vi "GetInstance.vi"(8 "error in (no error)":errorcluster, 11 "Singleton in":refnum<class "Singleton.lvclass">) -> (0 "error out":errorcluster, 3 "Singleton out":refnum<class "Singleton.lvclass">)   [LabVIEW 2014]
uses:
  Singleton.lvclass
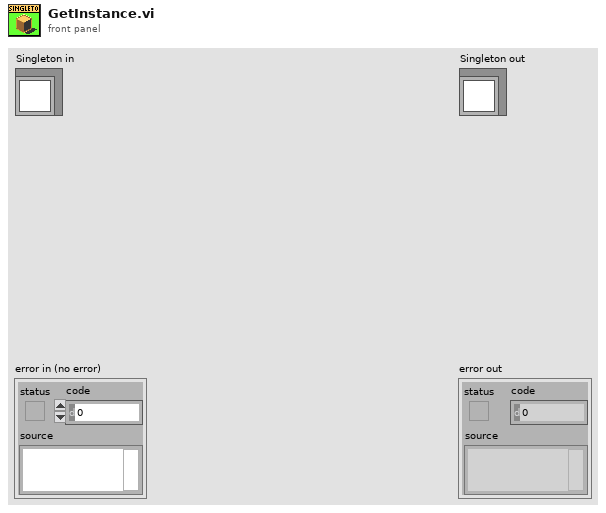
[diagram p1: front panel]
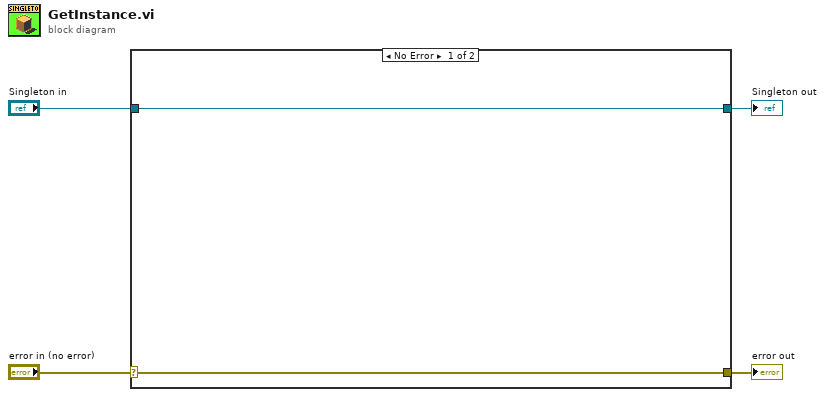
[diagram p0: block diagram]
diagram:
  n1 = case shown="No Error" "error in (no error)" {
    selector: "error in (no error)" -> [w5 w8]
    tunnel: [w5 w8] -> w3
    tunnel: [w6 w7] -> w1
    tunnel: "Singleton in" -> [w6 w7]
    frame No Error {
    }
    frame Error {
    }
  }
  "error out" <- w3
  "Singleton out" <- w1
